vi "Build.vi"(9 "XYZTheta":dbl[](array[numeric]), 10 "Pattern Coordinates":dbl[][](array[numeric]), 11 "Dispense Offset in":refnum<class "Dispense Offset.lvclass">) -> (1 "Starting Coordinates":dbl[](array[numeric]), 3 "Dispense Offset out":refnum<class "Dispense Offset.lvclass">)   [LabVIEW 2019, in "Dispense Offset.lvclass"]
uses:
  Dispense Offset.lvclass
  Dispense Offset.lvclass/Dispense Offset.ctl
  <vilib>/Analysis/coordinate.llb/2D Cartesian Coordinate Rotation (Scalar).vi
  <vilib>/Analysis/NI_AALPro.lvlib
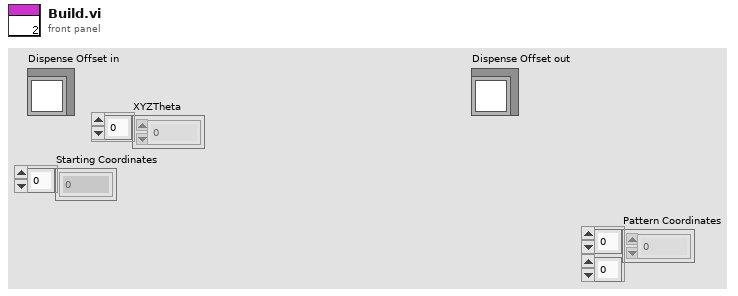
[diagram p1: front panel]
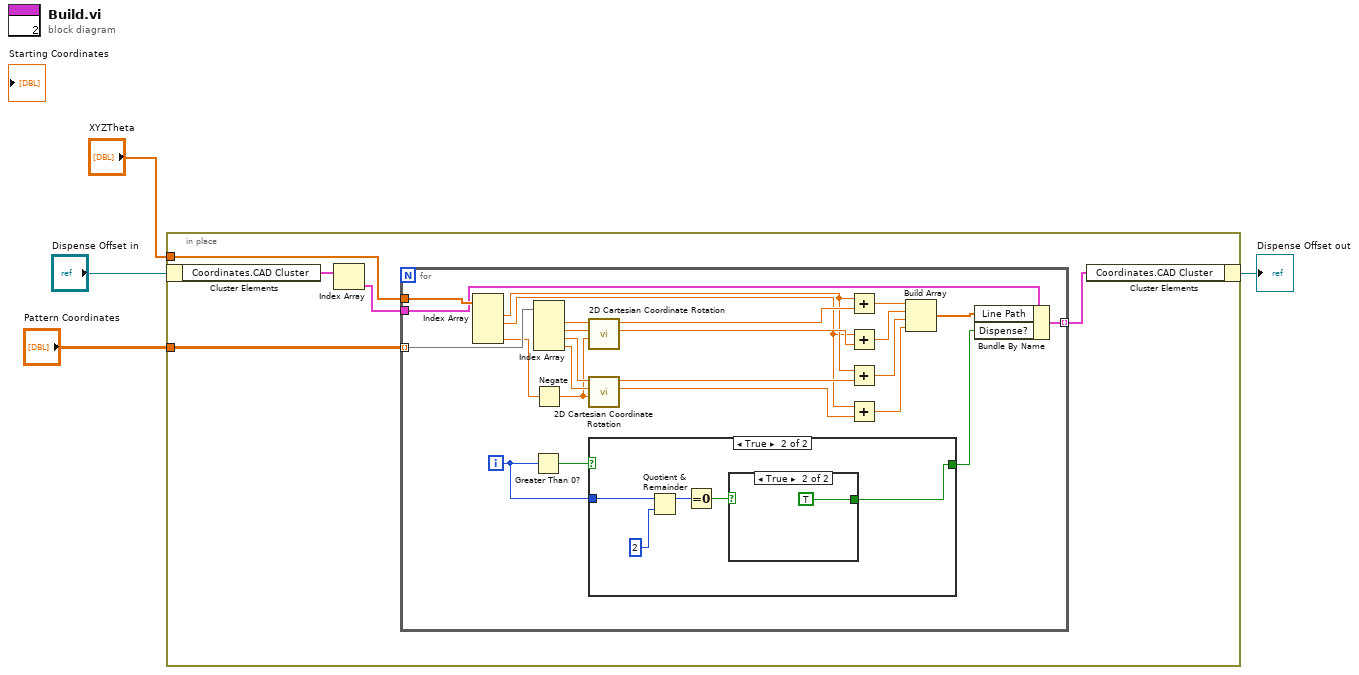
[diagram p0: block diagram]
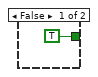
[diagram p2: hidden frame]
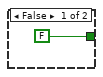
[diagram p3: hidden frame]
diagram:
  n1 = in-place {
    in-place-border: "Pattern Coordinates" -> [w9]
    in-place-border: "XYZTheta" -> [w8]
    n2 = in-place-cluster #1("Dispense Offset in") -> ("Coordinates.CAD Cluster"=w7:cluster{"Dispense?":bool, "Line Path":dbl[]}[])
    n3 = Index Array(array=w7) -> (element=w6:cluster{"Dispense?":bool, "Line Path":dbl[]})  [unwired: 1 in]
    n4 = for {
      tunnel: w9 -> [w33] mode=indexing
      tunnel: w8 -> [w32]
      tunnel: w6 -> [w15]
      tunnel: [w14] -> w5 mode=indexing
      i -> [w10]
      n5 = Index Array(array=w32) -> (element #1=w21:dbl, element #2=w19:dbl, element #4=w31:dbl)  [unwired: 4 in, 1 out]
      n6 = Greater Than 0?(x=w10) -> (x > 0?=w12:bool)
      n7 = Index Array(array=w33) -> (element #1=w30:dbl, element #2=w29:dbl, element #3=w28:dbl, element #4=w27:dbl)  [unwired: 4 in]
      n8 = Negate(x=w31) -> (-x=w26:dbl)
      n9 = call-poly <vilib>:"2D Cartesian Coordinate Rotation.vi"("theta"=w26, "y"=w29, "x"=w30) -> ("y out"=w24:dbl, "x out"=w25:dbl)  [unwired: 6 in, 1 out]
      n10 = call-poly <vilib>:"2D Cartesian Coordinate Rotation.vi"("theta"=w26, "y"=w27, "x"=w28) -> ("y out"=w18:dbl, "x out"=w20:dbl)  [unwired: 6 in, 1 out]
      n11 = case shown="True" w12 {
        tunnel: [TRUE w36] -> w11
        tunnel: w10 -> [_ w38]
        frame False {
        }
        frame True {
          n12 = Quotient & Remainder(x=w38, y=2) -> (x-y*floor(x/y)=w39:i32)  [unwired: 1 out]
          n13 = Equal To 0?(x=w39) -> (x = 0?=w37:bool)
          n14 = case shown="True" w37 {
            tunnel: [FALSE TRUE] -> w36
            frame False {
            }
            frame True {
            }
          }
        }
      }
      n15 = Add(x=w21, y=w25) -> (x+y=w23:dbl)
      n16 = Add(x=w19, y=w24) -> (x+y=w22:dbl)
      n17 = Add(x=w21, y=w20) -> (x+y=w17:dbl)
      n18 = Add(x=w19, y=w18) -> (x+y=w16:dbl)
      n19 = Build Array(w23, w22, w17, w16) -> (w13:dbl[])
      n20 = Bundle By Name(cluster=w15, "Line Path"=w13, "Dispense?"=w11) -> (w14:cluster{"Dispense?":bool, "Line Path":dbl[]})
    }
    n21 = in-place-cluster #1("Coordinates.CAD Cluster"=w5) -> (→"Dispense Offset out":refnum<class "Dispense Offset.lvclass">)
  }
